vi "Get Wheel Parameter by Name.vi"(8 "error in (no error)":errorcluster, 10 "parameter name":string, 11 "wheel in":refnum<class "NI_Robotics_Steering Wheel.lvclass">) -> (0 "error out":errorcluster, 1 "found?":bool, 2 "parameter value":variant, 3 "wheel out":refnum<class "NI_Robotics_Steering Wheel.lvclass">)   [LabVIEW 2017, in "NI_Robotics_Steering Wheel.lvclass"]
uses:
  <vilib>/robotics/Steering/Steering Wheel/NI_Robotics_Steering Wheel.lvclass
  <vilib>/robotics/Steering/Steering Wheel/NI_Robotics_Steering Wheel.lvclass/NI_Robotics_Steering Wheel.ctl
  <vilib>/robotics/Steering/Wheel/NI_Robotics_Wheel.lvclass
  <vilib>/robotics/Actuation/Motor Communication/NI_Robotics_Motor Communication.lvclass
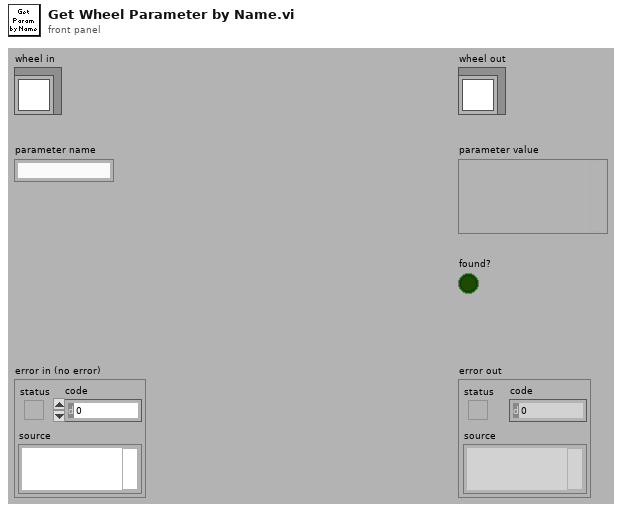
[diagram p1: front panel]
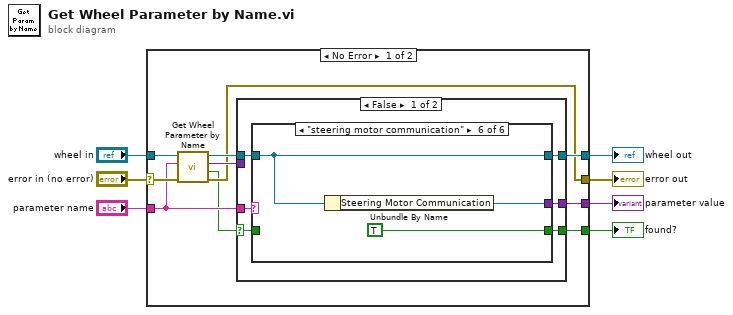
[diagram p0: block diagram]
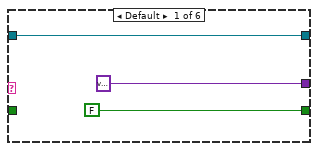
[diagram p2: hidden frame]
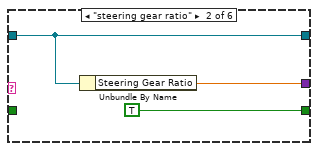
[diagram p3: hidden frame]
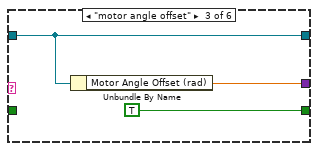
[diagram p4: hidden frame]
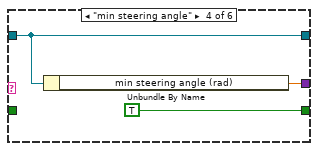
[diagram p5: hidden frame]
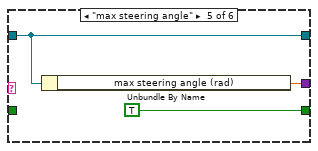
[diagram p6: hidden frame]
diagram:
  n1 = case shown="No Error" "error in (no error)" {
    selector: "error in (no error)" -> [w16 w45]
    tunnel: [w10 w45] -> w7
    tunnel: [w8 _] -> w6
    tunnel: [w12 _] -> w5
    tunnel: [w13 w46] -> w4
    tunnel: "parameter name" -> [w11 _]
    tunnel: "wheel in" -> [w17 w46]
    frame No Error {
      n2 = call-parent "Get Wheel Parameter by Name.vi"("error in (no error)"=w16, "parameter name"=w11, "wheel in"=w17) -> ("error out"=w10:errorcluster, "found?"=w9:bool, "parameter value"=w15:variant, "wheel out"=w14:refnum<class "NI_Robotics_Steering Wheel.lvclass">)  [unwired: 5 in]
      n3 = case shown="False" w9 {
        selector: w9 -> [w19 w42]
        tunnel: w15 -> [_ w43]
        tunnel: w14 -> [w23 w44]
        tunnel: [w21 w44] -> w13
        tunnel: [w20 w43] -> w12
        tunnel: w11 -> [w22 _]
        tunnel: [w18 w42] -> w8
        frame False {
          n4 = case shown="\"steering motor communication\"" w22 {
            tunnel: w23 -> [w26 w28 w31 w34 w37 w40]
            tunnel: [w26 w28 w31 w34 w37 w40] -> w21
            tunnel: [variant ("parameter value") w29 w32 w35 w38 w41] -> w20
            tunnel: w19 -> [_ _ _ _ _ _]
            tunnel: [FALSE TRUE TRUE TRUE TRUE TRUE] -> w18
            frame Default {
            }
            frame "steering gear ratio" {
              n5 = Unbundle By Name(w28) -> ("Steering Gear Ratio"=w29:dbl)
            }
            frame "motor angle offset" {
              n6 = Unbundle By Name(w31) -> ("Motor Angle Offset (rad)"=w32:dbl)
            }
            frame "min steering angle" {
              n7 = Unbundle By Name(w34) -> ("min steering angle (rad)"=w35:dbl)
            }
            frame "max steering angle" {
              n8 = Unbundle By Name(w37) -> ("max steering angle (rad)"=w38:dbl)
            }
            frame "steering motor communication" {
              n9 = Unbundle By Name(w40) -> ("Steering Motor Communication"=w41:refnum<class "NI_Robotics_Motor Communication.lvclass">)
            }
          }
        }
        frame True {
        }
      }
    }
    frame Error {
    }
  }
  "error out" <- w7
  "wheel out" <- w4
  "parameter value" <- w5
  "found?" <- w6
